vi "Measure Procedure.vi"(8 "error in":errorcluster, 9 "fileName":string, 10 "Request for procedure":enum16{"State", "Save", "Abort", "Start"}(ring), 11 "LoadProcedure":refnum<k24>) -> (0 "error out":errorcluster, 1 "IsMeasuring":bool)   [LabVIEW 2011]
doc: "To start, abort and save a measurement."
uses:
  C:/Program Files/Metrohm Autolab/Autolab SDK 1.10/EcoChemie.Autolab.Sdk.dll
  EcoChemie.Autolab.Sdk.dll
panel:
  in  "Stop":bool
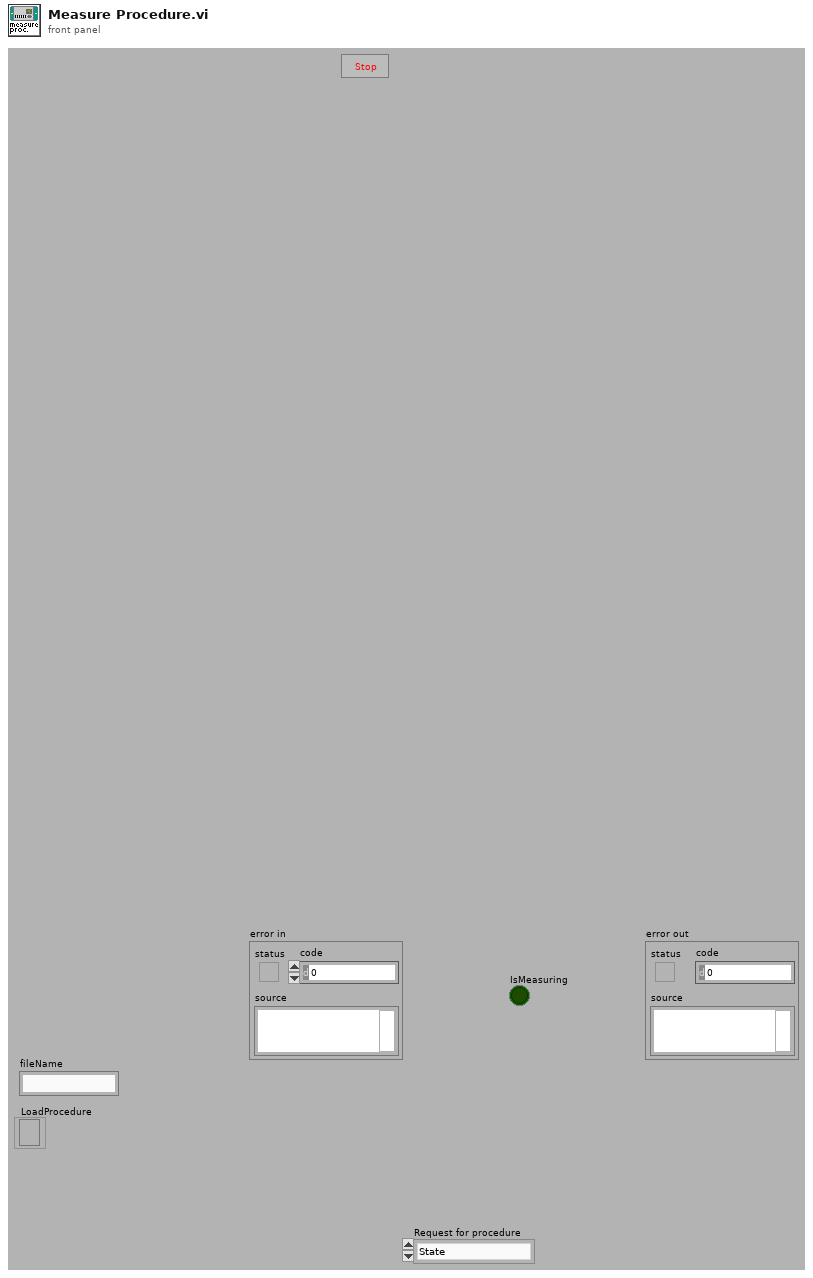
[diagram p1: front panel]
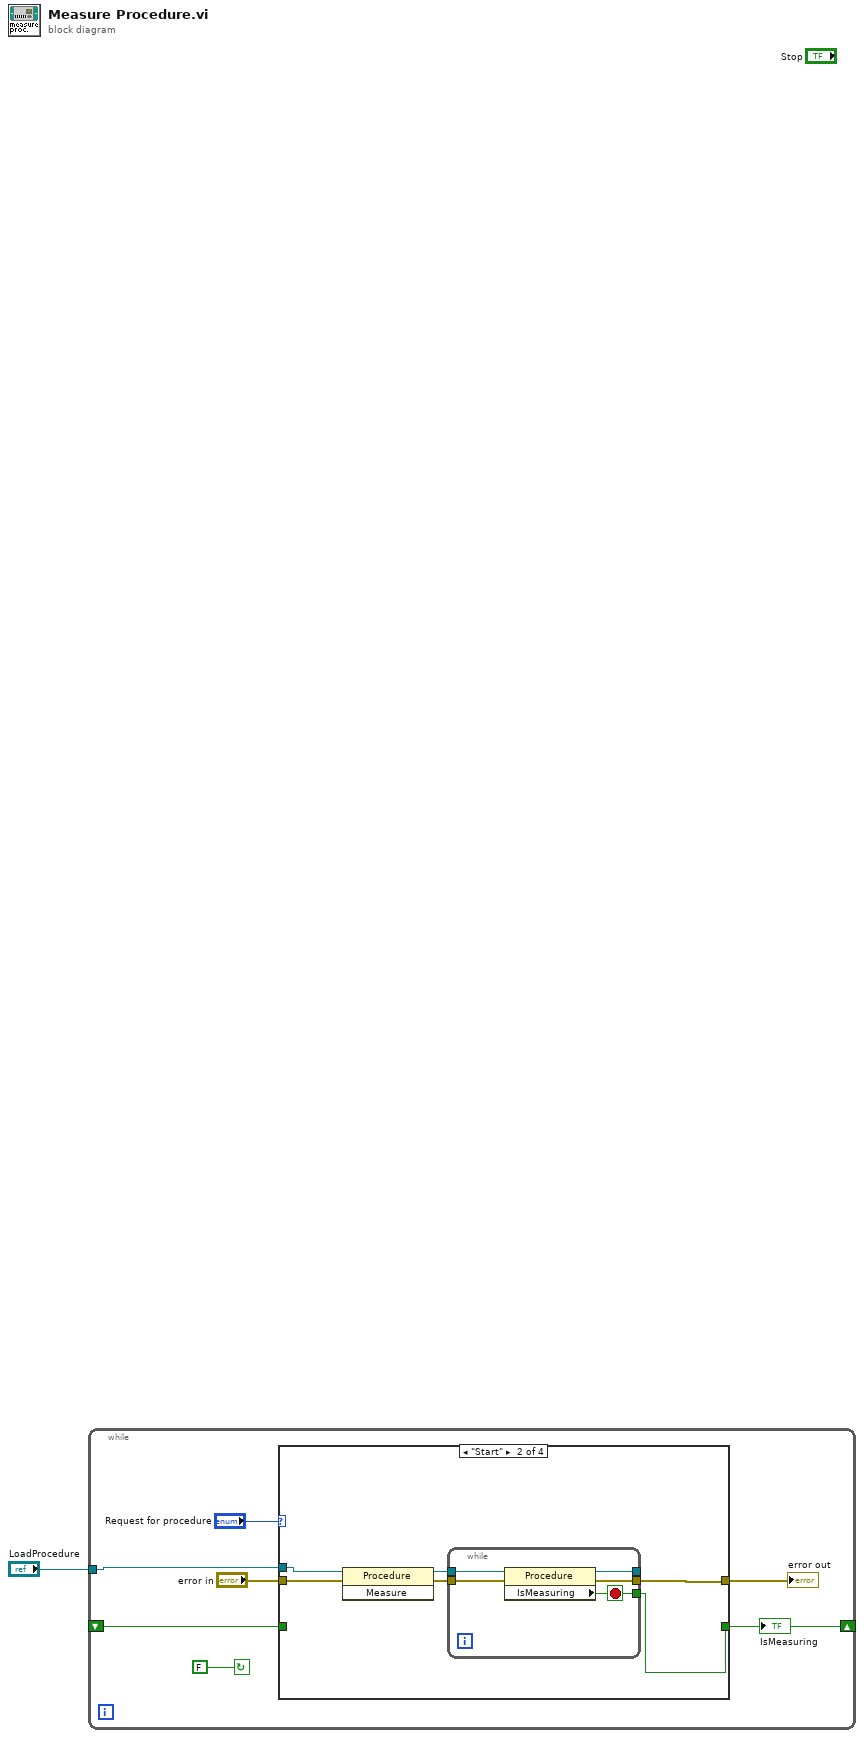
[diagram p0: block diagram]
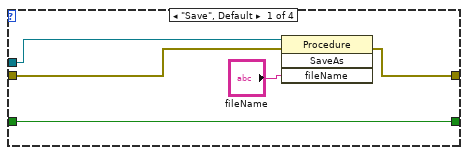
[diagram p2: hidden frame]
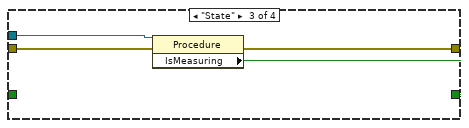
[diagram p3: hidden frame]
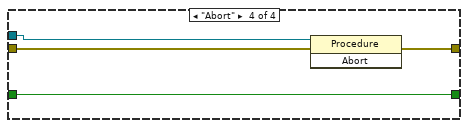
[diagram p4: hidden frame]
diagram:
  n1 = while {
    shift-right: [w4] -> _
    shift-left: _ -> [w5]
    tunnel: "LoadProcedure" -> [w2]
    stop <- FALSE continue-if-true
    n2 = case shown="\"Start\"" "Request for procedure" {
      tunnel: "error in" -> [w12 w16 w28 w32]
      tunnel: [w11 w18 w27 w31] -> w3
      tunnel: [w13 w19 w26 w30] -> w4
      tunnel: w5 -> [w13 _ _ w30]
      tunnel: w2 -> [w9 w17 w25 w29]
      frame "Save", Default {
        n3 = invoke class="Procedure" method="SaveAs"(reference=w9, error in=w12, "fileName"="fileName") -> (error out=w11:errorcluster)  [unwired: 1 in, 3 out]
      }
      frame "Start" {
        n4 = invoke class="Procedure" method="Measure"(reference=w17, error in=w16) -> (reference out=w14:refnum<k24>, error out=w15:errorcluster)  [unwired: 1 in, 1 out]
        n5 = while {
          tunnel: [w24] -> _
          tunnel: [w23] -> w18
          tunnel: [w22] -> w19
          tunnel: w15 -> [w21]
          tunnel: w14 -> [w20]
          stop <- w22 stop-if-true
          n6 = property class="Procedure"(reference=w20, error in=w21) -> (reference out=w24:refnum<k24>, error out=w23:errorcluster, "IsMeasuring"=w22:bool)
        }
      }
      frame "State" {
        n7 = property class="Procedure"(reference=w25, error in=w28) -> (error out=w27:errorcluster, "IsMeasuring"=w26:bool)  [unwired: 1 out]
      }
      frame "Abort" {
        n8 = invoke class="Procedure" method="Abort"(reference=w29, error in=w32) -> (error out=w31:errorcluster)  [unwired: 1 in, 2 out]
      }
    }
    "error out" <- w3
    "IsMeasuring" <- w4
  }
